vi "Data Check.vi"(0 "RFFE Extended Command in":refnum<class "RFFE Extended Command.lvclass">, 11 "error in (no error)":errorcluster) -> (4 "RFFE Extended Command out":refnum<class "RFFE Extended Command.lvclass">, 15 "error out":errorcluster)   [LabVIEW 2018, in "MIPI RFFE API.lvlib" / "RFFE Extended Command.lvclass"]
uses:
  RFFE Extended Command.lvclass
  Get Byte Count Limit.vi
  Command/RFFE Command.lvclass
  MIPI RFFE API.lvlib
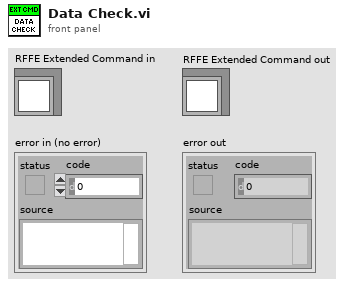
[diagram p1: front panel]
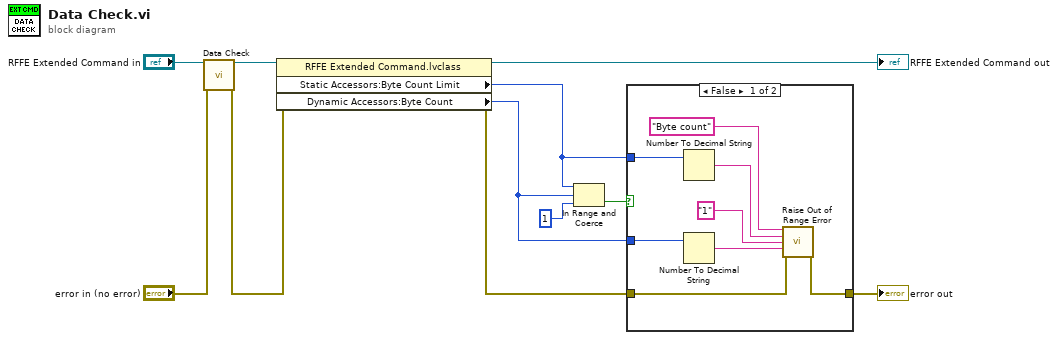
[diagram p0: block diagram]
diagram:
  n1 = call-parent "Data Check.vi"("RFFE Command in"="RFFE Extended Command in", "error in (no error)"="error in (no error)") -> ("RFFE Command out"=w8:refnum<class "RFFE Extended Command.lvclass">, "error out"=w7:errorcluster)  [unwired: 12 in]
  n2 = property class="RFFE Extended Command.lvclass"(reference=w8, error in=w7) -> (reference out=→"RFFE Extended Command out":refnum<class "RFFE Extended Command.lvclass">, error out=w5:errorcluster, "Static Accessors:Byte Count Limit"=w1:i32, "Dynamic Accessors:Byte Count"=w4:i32)
  n3 = In Range and Coerce(upper limit=w1, x=w4, lower limit=1) -> (In Range?=w2:bool)  [unwired: 1 out]
  n4 = case shown="False" w2 {
    tunnel: w5 -> [w19 w20]
    tunnel: [w13 w20] -> w9
    tunnel: w4 -> [w15 _]
    tunnel: w1 -> [w17 _]
    frame False {
      n5 = Number To Decimal String(number=w17) -> (decimal integer string=w16:string)  [unwired: 1 in]
      n6 = Number To Decimal String(number=w15) -> (decimal integer string=w14:string)  [unwired: 1 in]
      n7 = call "Raise Out of Range Error.vi"("Parameter Name"="Byte count", "Upper Limit"=w16, "Lower Limit"="1", "As Found"=w14, "error in (no error)"=w19) -> ("error out"=w13:errorcluster)  [unwired: 10 in]
    }
    frame True {
    }
  }
  "error out" <- w9
